vi "file list -- accumulate V3.vi"(11 "file path":path=path "/snowfall/Users/arcadi/Desktop/Ultrasound/Experiment/YBCO_4/Round1/Sweep12/June_2011/062511/221.16400K_300_3100_001_062511.dat") -> (0 "timestamp":dbl[](array[numeric]), 2 "sweep file name array":T1[](array[typedef]), 3 "temperatures":dbl[](array[numeric]))   [LabVIEW 2010]
uses:
  sweep file name.ctl
panel:
  in  "dummy 2":T1={"temperature"=0.0, "temperature str"="", "file path"=path "/snowfall/Users/arcadi/Desktop/Ultrasound/Experiment/YBCO_4/Round1/Sweep12/June_2011/062511/221.16400K_300_3100_001_062511.dat", "last mod"=timestamp(0 s since 1904-01-01), "file name str"="", "mod time(min)"=0.0, "file format"=enum.""}
  in  "sweep file name":T1={"temperature"=0.0, "temperature str"="", "file path"=path "/snowfall/Users/arcadi/Desktop/Ultrasound/Experiment/YBCO_4/Round1/Sweep12/June_2011/062511/221.16400K_300_3100_001_062511.dat", "last mod"=timestamp(0 s since 1904-01-01), "file name str"="", "mod time(min)"=0.0, "file format"=enum.""}
  in  "dummy":T1={"temperature"=0.0, "temperature str"="", "file path"=path "/snowfall/Users/arcadi/Desktop/Ultrasound/Experiment/YBCO_4/Round1/Sweep12/June_2011/062511/221.16400K_300_3100_001_062511.dat", "last mod"=timestamp(0 s since 1904-01-01), "file name str"="", "mod time(min)"=0.0, "file format"=enum.""}
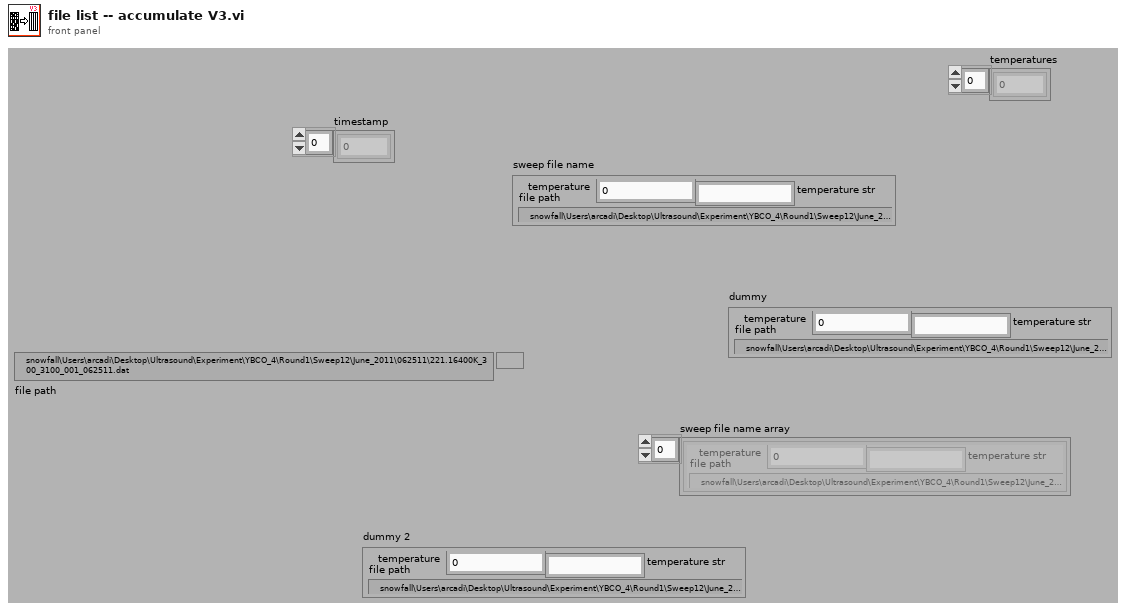
[diagram p1: front panel]
types:
  T1 = typedef "sweep file name.ctl" = cluster{"temperature":dbl, "temperature str":string, "file path":path, "last mod":timestamp, "file name str":string, "mod time(min)":dbl, "file format":enum16{"", "ascii", "binary"}}
  T2 = cluster{"basename":string, "dat":bool, "bin":bool}
  T3 = cluster{"basename":string, "dat":bool, "bin":bool}[]
  T4 = cluster{"temperature":string, "from F":string, "to F":string, "counter":string, "date":string}
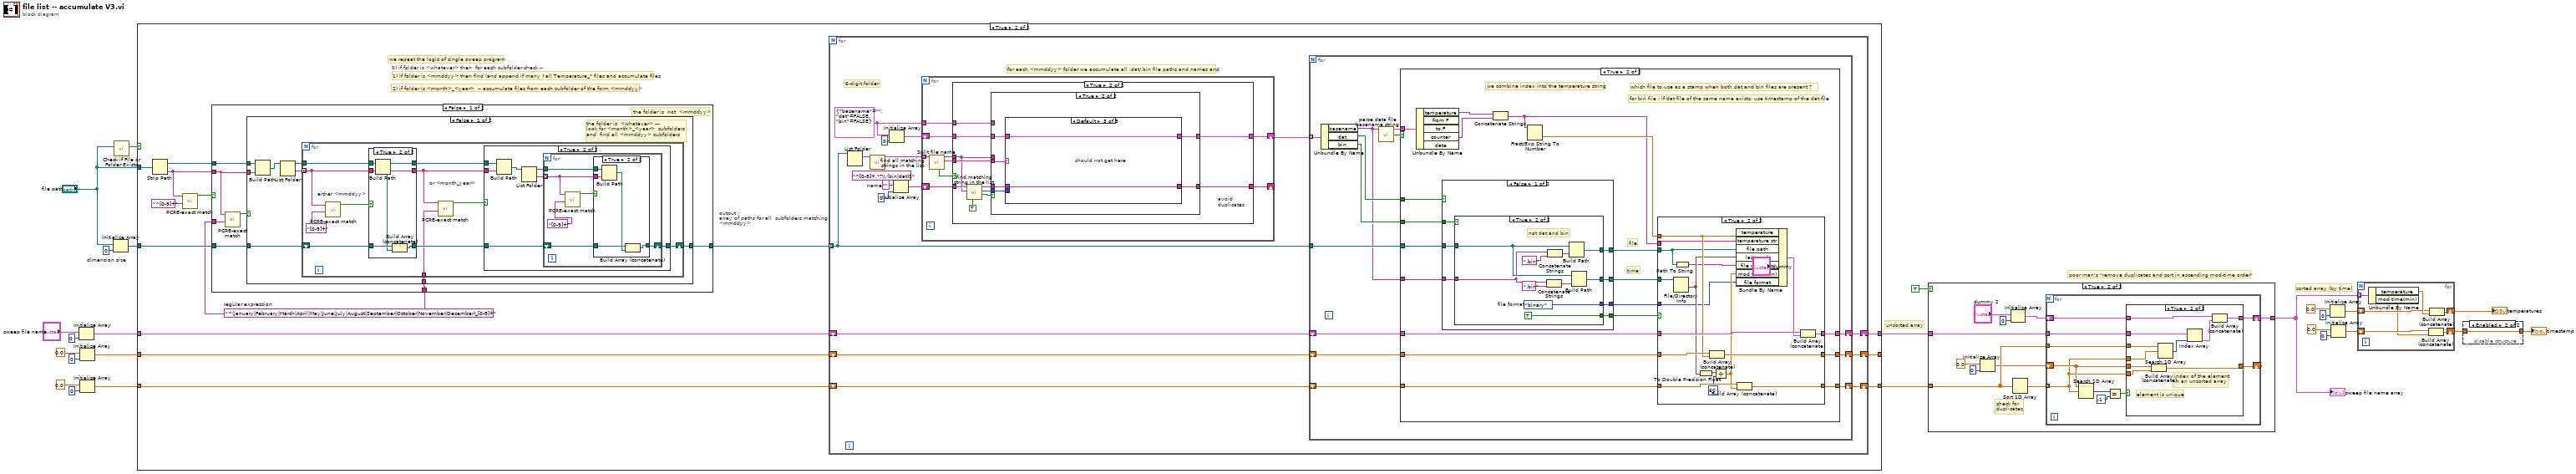
[diagram p0: block diagram]
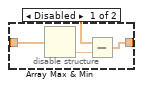
[diagram p2: hidden frame]
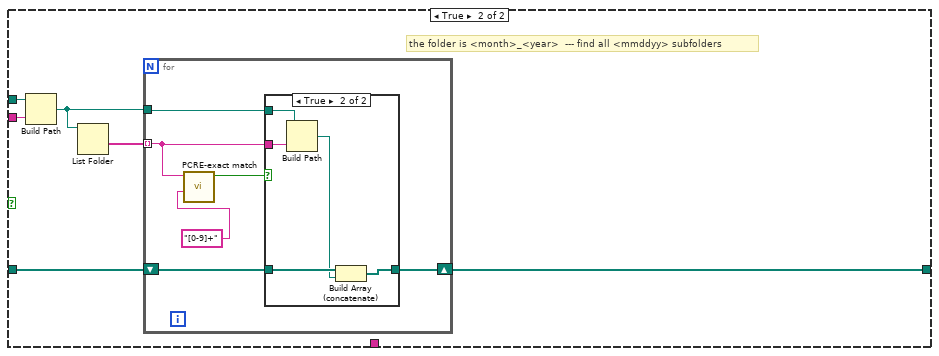
[diagram p9: hidden frame]
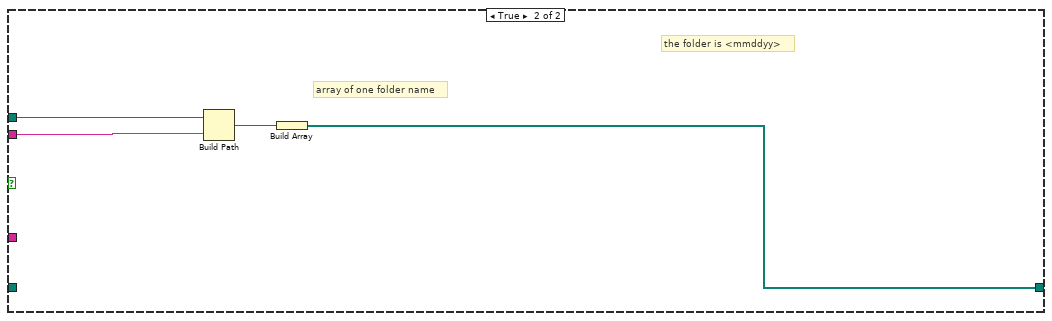
[diagram p11: hidden frame]
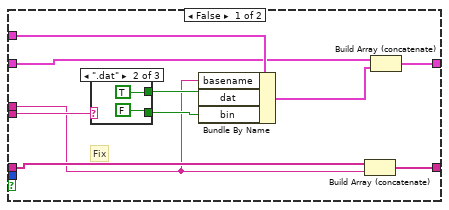
[diagram p13: hidden frame]
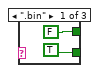
[diagram p14: hidden frame]
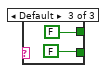
[diagram p15: hidden frame]
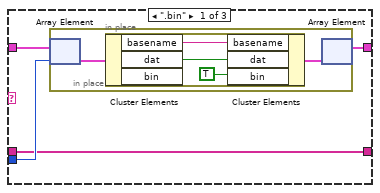
[diagram p16: hidden frame]
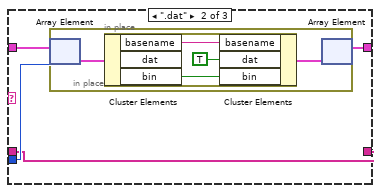
[diagram p17: hidden frame]
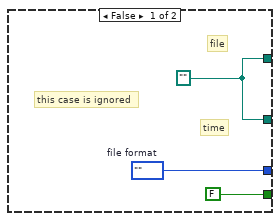
[diagram p20: hidden frame]
diagram:
  w3 = 0  # dimension size
  # "sorted array (by time)"
  # "unsorted array"
  # "poor man's \"remove duplicates and sort in ascending mod-time order\""
  n1 = Initialize Array("sweep file name", 0 ("dimension size")) -> (w21:T1[])
  n2 = Initialize Array(0.0 ("dimension size"), 0 ("dimension size")) -> (w20:dbl[])
  n3 = Initialize Array(0.0 ("dimension size"), 0 ("dimension size")) -> (w17:dbl[])
  n4 = Initialize Array("file path", w3) -> (w1:path[])
  n5 = call <vilib>:"Check if File or Folder Exists.vi"("path"="file path") -> ("file or folder exists?"=w26:bool)  [unwired: 8 in, 2 out]
  n6 = case shown="True" w26 {
    tunnel: "file path" -> [_ w39]
    tunnel: [w29 w41] -> w14
    tunnel: [w28 w40] -> _
    tunnel: w21 -> [w29 w43]
    tunnel: w20 -> [w28 w42]
    tunnel: w17 -> [w27 w38]
    tunnel: [w27 w37] -> w15
    tunnel: w1 -> [_ w34]
    frame False {
    }
    frame True {
      w33 = "^(January|February|March|April|May|June|July|August|September|October|November|December)_[0-9]+"  # regular expression
      # "0) if folder is <whatever> then  for each subfolder check --"
      # "1) if folder is <mmddyy> then find (and append if many ) all Temperature_* files and accumulate files"
      # "2) if folder is <month>_<year>  -- accumulate files from each subfolder of the form <mmddyy>"
      # "we repeat the logic of single sweep program"
      # "output : \narray of paths for all  subfolders matching  <mmddyy>"
      n7 = Strip Path(path=w39) -> (stripped path=w36:path, name=w32:string)
      n8 = call "PCRE-exact match.vi"("regular expression"="^[0-9]+", "input string"=w32) -> ("exact match"=w30:bool)  [unwired: 8 in, 1 out]
      n9 = case shown="False" w30 {
        tunnel: [w50 w118] -> w35
        tunnel: w36 -> [w49 w117]
        tunnel: w32 -> [w45 w116]
        tunnel: w33 -> [w46 _]
        tunnel: w34 -> [w48 _]
        tunnel: w33 -> [w47 _]
        frame False {
          # "the folder is  not  <mmddyy>"
          n10 = call "PCRE-exact match.vi"("regular expression"=w46, "input string"=w45) -> ("exact match"=w44:bool)  [unwired: 8 in, 1 out]
          n11 = case shown="False" w44 {
            tunnel: [w52 w101] -> w50
            tunnel: w45 -> [w55 w100]
            tunnel: w49 -> [w56 w99]
            tunnel: w48 -> [w54 w98]
            tunnel: w47 -> [w53 _]
            frame False {
              # "the folder is  <whatever> --- \nlook for <month>_<year>  subfolders \nand  find all <mmddyy> subfolders"
              n12 = Build Path(base path=w56, name or relative path=w55) -> (appended path=w57:path)
              n13 = List Folder(path=w57) -> (path out=w51:path, folder names=w58:string[])  [unwired: 3 in, 2 out]
              n14 = for {
                tunnel: w58 -> [w64] mode=indexing
                shift-right: [w68] -> w52
                shift-left: w54 -> [w69]
                tunnel: w51 -> [w66]
                tunnel: w53 -> [w60]
                # "or <month_year>"
                # "either <mmddyy>"
                n15 = call "PCRE-exact match.vi"("regular expression"="[0-9]+", "input string"=w64) -> ("exact match"=w62:bool)  [unwired: 8 in, 1 out]
                n16 = case shown="True" w62 {
                  tunnel: w66 -> [w90 w93]
                  tunnel: w64 -> [w91 w94]
                  tunnel: w69 -> [w92 w97]
                  tunnel: [w92 w95] -> w67
                  tunnel: [w91 w94] -> w61
                  tunnel: [w90 w93] -> w65
                  frame False {
                  }
                  frame True {
                    n17 = Build Path(base path=w93, name or relative path=w94) -> (appended path=w96:path)
                    n18 = Build Array (concatenate)(w97, w96) -> (w95:path[])
                  }
                }
                n19 = call "PCRE-exact match.vi"("regular expression"=w60, "input string"=w61) -> ("exact match"=w59:bool)  [unwired: 8 in, 1 out]
                n20 = case shown="True" w59 {
                  tunnel: [w70 w73] -> w68
                  tunnel: w67 -> [w70 w74]
                  tunnel: w65 -> [_ w77]
                  tunnel: w61 -> [_ w76]
                  frame False {
                  }
                  frame True {
                    n21 = Build Path(base path=w77, name or relative path=w76) -> (appended path=w72:path)
                    n22 = List Folder(path=w72) -> (path out=w71:path, folder names=w75:string[])  [unwired: 3 in, 2 out]
                    n23 = for {
                      tunnel: w75 -> [w80] mode=indexing
                      shift-right: [w82] -> w73
                      shift-left: w74 -> [w83]
                      tunnel: w71 -> [w81]
                      n24 = call "PCRE-exact match.vi"("regular expression"="[0-9]+", "input string"=w80) -> ("exact match"=w78:bool)  [unwired: 8 in, 1 out]
                      n25 = case shown="True" w78 {
                        tunnel: w83 -> [w84 w88]
                        tunnel: [w84 w87] -> w82
                        tunnel: w81 -> [_ w86]
                        tunnel: w80 -> [_ w85]
                        frame False {
                        }
                        frame True {
                          n26 = Build Path(base path=w86, name or relative path=w85) -> (appended path=w89:path)
                          n27 = Build Array (concatenate)(w88, w89) -> (w87:path[])
                        }
                      }
                    }
                  }
                }
              }
            }
            frame True {
              # "the folder is <month>_<year>  --- find all <mmddyy> subfolders"
              n28 = Build Path(base path=w99, name or relative path=w100) -> (appended path=w102:path)
              n29 = List Folder(path=w102) -> (folder names=w103:string[])  [unwired: 3 in, 3 out]
              n30 = for {
                tunnel: w103 -> [w106] mode=indexing
                shift-right: [w107] -> w101
                shift-left: w98 -> [w108]
                tunnel: w102 -> [w109]
                n31 = call "PCRE-exact match.vi"("regular expression"="[0-9]+", "input string"=w106) -> ("exact match"=w104:bool)  [unwired: 8 in, 1 out]
                n32 = case shown="True" w104 {
                  tunnel: w109 -> [_ w115]
                  tunnel: w106 -> [_ w114]
                  tunnel: w108 -> [w110 w113]
                  tunnel: [w110 w111] -> w107
                  frame False {
                  }
                  frame True {
                    n33 = Build Path(base path=w115, name or relative path=w114) -> (appended path=w112:path)
                    n34 = Build Array (concatenate)(w113, w112) -> (w111:path[])
                  }
                }
              }
            }
          }
        }
        frame True {
          # "the folder is <mmddyy>"
          # "array of one folder name"
          n35 = Build Path(base path=w117, name or relative path=w116) -> (appended path=w119:path)
          n36 = Build Array(w119) -> (w118:path[])
        }
      }
      n37 = for {
        tunnel: w35 -> [w130] mode=indexing
        shift-right: [w134] -> w41
        shift-left: w43 -> [w136]
        shift-right: [w135] -> w40
        shift-left: w42 -> [w133]
        shift-right: [w131] -> w37
        shift-left: w38 -> [w132]
        w120 = T2 {"basename"="", "dat"=FALSE, "bin"=FALSE}
        w124 = ""  # name
        # "6-digit folder"
        # "for each <mmddyy> folder we accumulate all .dat/.bin file paths and names and"
        n38 = List Folder(path=w130) -> (filenames=w129:string[])  [unwired: 3 in, 3 out]
        n39 = call "find all matching strings in the list.vi"("regular expression"="^[0-9]+.*?\\.(bin|dat)$" ("pattern"), "strings"=w129) -> ("list of matching strings"=w127:string[])  [unwired: 7 in, 2 out]
        n40 = Initialize Array(w120, 0) -> (w122:T3)
        n41 = Initialize Array(w124, 0) -> (w123:string[])
        n42 = for {
          tunnel: w127 -> [w145] mode=indexing
          shift-right: [w141] -> _
          shift-left: w123 -> [w140]
          shift-right: [w142] -> w121
          shift-left: w122 -> [w144]
          tunnel: w120 -> [w139]
          n43 = call "Split file name.vi"("file name"=w145) -> ("extension"=w143:string, "name"=w138:string, "exact match"=w137:bool)  [unwired: 8 in]
          n44 = case shown="True" w137 {
            tunnel: w144 -> [w147 w155]
            tunnel: w143 -> [_ w154]
            tunnel: [w147 w152] -> w142
            tunnel: [w146 w151] -> w141
            tunnel: w140 -> [w146 w150]
            tunnel: w139 -> [_ w149]
            tunnel: w138 -> [_ w148]
            frame False {
            }
            frame True {
              # "avoid \nduplicates"
              n45 = call "find matching string in the list.vi"("quote specials"=TRUE, "regular expression"=w148, "strings"=w150) -> ("match found"=w156:bool, "matching string index"=w153:i32)  [unwired: 6 in, 1 out]
              n46 = case shown="True" w156 {
                tunnel: w155 -> [w161 w179]
                tunnel: w154 -> [w164 w178]
                tunnel: w153 -> [_ w177]
                tunnel: [w159 w176] -> w152
                tunnel: [w166 w175] -> w151
                tunnel: w150 -> [w167 w174]
                tunnel: w148 -> [w158 _]
                tunnel: w149 -> [w165 _]
                frame False {
                  # "Fix"
                  n47 = case shown="\".dat\"" w164 {
                    tunnel: [FALSE ("quote specials") TRUE ("quote specials") FALSE ("quote specials")] -> w163
                    tunnel: [TRUE ("quote specials") FALSE ("quote specials") FALSE ("quote specials")] -> w162
                    frame ".bin" {
                    }
                    frame ".dat" {
                    }
                    frame Default {
                    }
                  }
                  n48 = Bundle By Name(cluster=w165, "basename"=w158, "dat"=w163, "bin"=w162) -> (w160:T2)
                  n49 = Build Array (concatenate)(w167, w158) -> (w166:string[])
                  n50 = Build Array (concatenate)(w161, w160) -> (w159:T3)
                }
                frame True {
                  n51 = case shown="Default" w178 {
                    tunnel: w179 -> [w183 w192 w199]
                    tunnel: w177 -> [w181 w191 _]
                    tunnel: [w182 w190 w199] -> w176
                    tunnel: [w180 w189 w198] -> w175
                    tunnel: w174 -> [w180 w189 w198]
                    frame ".bin" {
                      n52 = in-place {
                        n53 = in-place-array #1(w183, w181) -> (w185:T2)
                        n54 = in-place {
                          n55 = in-place-cluster #2(w185) -> ("basename"=w188:string, "dat"=w186:bool)  [unwired: 1 out]
                          n56 = in-place-cluster #2("basename"=w188, "dat"=w186, "bin"=TRUE ("quote specials")) -> (w184:T2)
                        }
                        n57 = in-place-array #1(w184) -> (w182:T3)  [unwired: 1 out]
                      }
                    }
                    frame ".dat" {
                      n58 = in-place {
                        n59 = in-place-array #3(w192, w191) -> (w194:T2)
                        n60 = in-place {
                          n61 = in-place-cluster #4(w194) -> ("basename"=w197:string, "bin"=w196:bool)  [unwired: 1 out]
                          n62 = in-place-cluster #4("basename"=w197, "dat"=TRUE ("quote specials"), "bin"=w196) -> (w193:T2)
                        }
                        n63 = in-place-array #3(w193) -> (w190:T3)  [unwired: 1 out]
                      }
                    }
                    frame Default {
                      # "should not get here"
                    }
                  }
                }
              }
            }
          }
        }
        n64 = for {
          tunnel: w121 -> [w205] mode=indexing
          tunnel: w130 -> [w212]
          shift-right: [w210] -> w134
          shift-left: w136 -> [w211]
          shift-right: [w208] -> w135
          shift-left: w133 -> [w209]
          shift-right: [w206] -> w131
          shift-left: w132 -> [w207]
          n65 = Unbundle By Name(w205) -> ("basename"=w200:string, "dat"=w202:bool, "bin"=w201:bool)
          n66 = call "parse data file basename string.vi"("base name"=w200) -> ("output cluster"=w203:T4, "exact match"=w204:bool)  [unwired: 9 in]
          n67 = case shown="True" w204 {
            tunnel: w212 -> [_ w222]
            tunnel: w211 -> [w215 w234]
            tunnel: [w215 w233] -> w210
            tunnel: w209 -> [w214 w232]
            tunnel: [w214 w231] -> w208
            tunnel: w207 -> [w213 w230]
            tunnel: [w213 w229] -> w206
            tunnel: w203 -> [_ w227]
            tunnel: w202 -> [_ w224]
            tunnel: w201 -> [_ w223]
            tunnel: w200 -> [_ w221]
            frame False {
            }
            frame True {
              # "file"
              # "time"
              # "we combine index into the temperature string"
              # "which file to use as a stamp when both dat and bin files are present ?"
              # "for bin file : if dat file of the same name exists, use timestamp of the dat file"
              n68 = Unbundle By Name(w227) -> ("temperature"=w226:string, "counter"=w225:string)  [unwired: 3 out]
              n69 = case shown="False" w224 {
                tunnel: w223 -> [w257 w282]
                tunnel: w222 -> [w259 w281]
                tunnel: w221 -> [w258 w280]
                tunnel: [w262 w279] -> w218
                tunnel: [w261 w278] -> w220
                tunnel: [w260 w277] -> w219
                tunnel: [w256 w276] -> w216
                frame False {
                  n70 = case shown="True" w257 {
                    tunnel: w259 -> [_ w271]
                    tunnel: w258 -> [_ w270]
                    tunnel: [w263 w274] -> w262
                    tunnel: [w263 w269] -> w261
                    tunnel: [w265 w267] -> w260
                    tunnel: [FALSE ("quote specials") TRUE ("quote specials")] -> w256
                    frame False {
                      w263 = path ""
                      w265 = enum16{"", "ascii", "binary"}.""  # file format
                      # "time"
                      # "file"
                      # "this case is ignored"
                    }
                    frame True {
                      w267 = enum16{"", "ascii", "binary"}."binary"  # file format
                      # "not dat and bin"
                      n71 = Concatenate Strings(w270, ".bin" ("string")) -> (w272:string)
                      n72 = Concatenate Strings(w270, ".bin" ("string")) -> (w268:string)
                      n73 = Build Path(base path=w271, name or relative path=w268) -> (appended path=w274:path)
                      n74 = Build Path(base path=w271, name or relative path=w272) -> (appended path=w269:path)
                    }
                  }
                }
                frame True {
                  n75 = case shown="False" w282 {
                    tunnel: w281 -> [w288 w298]
                    tunnel: w280 -> [w284 w297]
                    tunnel: [w287 w301] -> w279
                    tunnel: [w286 w296] -> w278
                    tunnel: [w285 w294] -> w277
                    tunnel: [TRUE ("quote specials") TRUE ("quote specials")] -> w276
                    frame False {
                      w285 = enum16{"", "ascii", "binary"}."ascii"  # file format
                      # "dat and no  bin"
                      n76 = Concatenate Strings(w284, ".dat" ("string")) -> (w289:string)
                      n77 = Concatenate Strings(w284, ".dat" ("string")) -> (w290:string)
                      n78 = Build Path(base path=w288, name or relative path=w290) -> (appended path=w286:path)
                      n79 = Build Path(base path=w288, name or relative path=w289) -> (appended path=w287:path)
                    }
                    frame True {
                      w294 = enum16{"", "ascii", "binary"}."binary"  # file format
                      # "both dat and bin"
                      n80 = Concatenate Strings(w297, ".dat" ("string")) -> (w299:string)
                      n81 = Concatenate Strings(w297, ".bin" ("string")) -> (w295:string)
                      n82 = Build Path(base path=w298, name or relative path=w295) -> (appended path=w301:path)
                      n83 = Build Path(base path=w298, name or relative path=w299) -> (appended path=w296:path)
                    }
                  }
                }
              }
              n84 = Concatenate Strings(w226, w225) -> (w217:string)
              n85 = Fract/Exp String To Number(string=w217) -> (number=w228:dbl)  [unwired: 3 in, 1 out]
              n86 = case shown="True" w216 {
                tunnel: w234 -> [w237 w255]
                tunnel: [w237 w254] -> w233
                tunnel: w232 -> [w236 w253]
                tunnel: [w236 w252] -> w231
                tunnel: w230 -> [w235 w251]
                tunnel: [w235 w250] -> w229
                tunnel: w228 -> [_ w247]
                tunnel: w220 -> [_ w242]
                tunnel: w219 -> [_ w241]
                tunnel: w218 -> [_ w240]
                tunnel: w217 -> [_ w238]
                frame False {
                }
                frame True {
                  n87 = File/Directory Info(path=w242) -> (last mod=w246:timestamp)  [unwired: 1 in, 6 out]
                  n88 = Path To String(path=w240) -> (string=w239:string)
                  n89 = To Double Precision Float(number=w246) -> (double precision float=w245:dbl)
                  n90 = Build Array (concatenate)(w253, w247) -> (w252:dbl[])
                  n91 = Divide(x=w245, y=60) -> (x/y=w243:dbl)
                  n92 = Bundle By Name(cluster="dummy", "temperature"=w247, "temperature str"=w238, "file path"=w240, "last mod"=w246, "file name str"=w239, "mod time(min)"=w243, "file format"=w241) -> (w248:T1)
                  n93 = Build Array (concatenate)(w251, w243) -> (w250:dbl[])
                  n94 = Build Array (concatenate)(w255, w248) -> (w254:T1[])
                }
              }
            }
          }
        }
      }
    }
  }
  n95 = case shown="True" TRUE {
    tunnel: w15 -> [_ w307]
    tunnel: w14 -> [w303 w312]
    tunnel: [w303 w311] -> w4
    frame False {
    }
    frame True {
      # "check for \nduplicates"
      n96 = Initialize Array(0.0 ("dimension size"), 0 ("dimension size")) -> (w304:dbl[])
      n97 = Initialize Array("dummy 2", 0 ("dimension size")) -> (w308:T1[])
      n98 = Sort 1D Array(array=w307) -> (sorted array=w313:dbl[])
      n99 = for {
        shift-right: [w320] -> w311
        shift-left: w308 -> [w319]
        shift-right: [w318] -> _
        shift-left: w304 -> [w317]
        tunnel: w313 -> [w314] mode=indexing
        tunnel: w307 -> [w316]
        tunnel: w312 -> [w315]
        n100 = Search 1D Array(1D array=w317, element=w314) -> (index of element=w323:i32)  [unwired: 1 in]
        n101 = Equal?(x=w323, y=-1) -> (x = y?=w321:bool)
        n102 = case shown="True" w321 {
          tunnel: [w325 w334] -> w320
          tunnel: w319 -> [w325 w335]
          tunnel: [w324 w326] -> w318
          tunnel: w317 -> [w324 w328]
          tunnel: w316 -> [_ w333]
          tunnel: w314 -> [_ w332]
          tunnel: w315 -> [_ w330]
          tunnel: w314 -> [_ w327]
          frame False {
            # "element is not unique"
          }
          frame True {
            # "index of the element \nin an unsorted array"
            # "element is unique"
            n103 = Build Array (concatenate)(w328, w327) -> (w326:dbl[])
            n104 = Search 1D Array(1D array=w333, element=w332) -> (index of element=w331:i32)  [unwired: 1 in]
            n105 = Index Array(array=w330, index=w331) -> (element=w329:T1)
            n106 = Build Array (concatenate)(w335, w329) -> (w334:T1[])
          }
        }
      }
    }
  }
  "sweep file name array" <- w4
  n107 = Initialize Array(0.0 ("dimension size"), 0 ("dimension size")) -> (w11:dbl[])
  n108 = Initialize Array(0.0 ("dimension size"), 0 ("dimension size")) -> (w8:dbl[])
  n109 = for {
    tunnel: w4 -> [w342] mode=indexing
    shift-right: [w336] -> w7
    shift-left: w11 -> [w340]
    shift-right: [w337] -> w6
    shift-left: w8 -> [w339]
    n110 = Unbundle By Name(w342) -> ("temperature"=w341:dbl, "mod time(min)"=w338:dbl)
    n111 = Build Array (concatenate)(w339, w338) -> (w337:dbl[])
    n112 = Build Array (concatenate)(w340, w341) -> (w336:dbl[])
  }
  "temperatures" <- w7
  n113 = disable-structure shown="Enabled" {
    disable-tunnel: w6 -> [w344 w346]
    disable-tunnel: [w343 w346] -> w5
    frame Disabled {
      n114 = Array Max & Min(array=w344) -> (min value=w345:dbl)  [unwired: 3 out]
      n115 = Subtract(x=w344, y=w345) -> (x-y=w343:dbl[])
    }
    frame Enabled {
    }
  }
  "timestamp" <- w5
